vi "PeriodTuningSine.vi"(10 "cfspont":dbl, 11 "cf_right":dbl) -> (0 "Negwave":dbl, 1 "Postwave":dbl, 2 "Period":dbl, 3 "Phase reset":dbl)   [LabVIEW 2016]
uses:
  <vilib>/measure/NI_MABase.lvlib
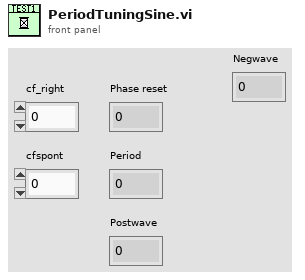
[diagram p1: front panel]
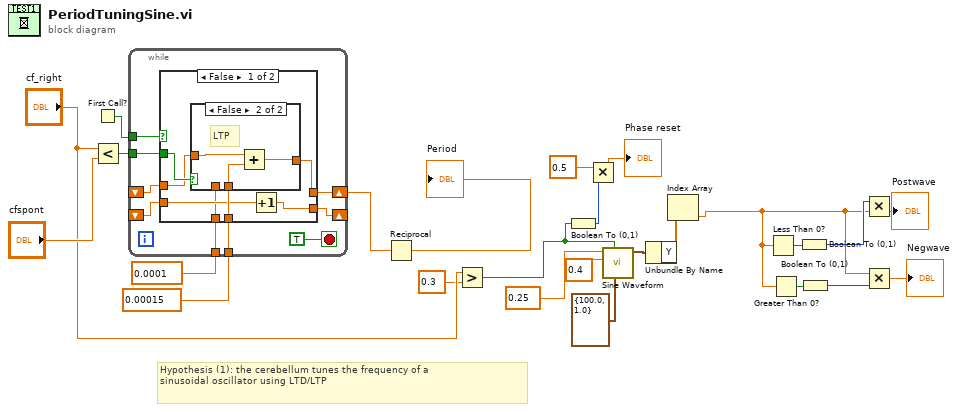
[diagram p0: block diagram]
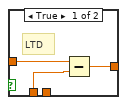
[diagram p2: hidden frame]
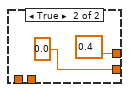
[diagram p3: hidden frame]
diagram:
  # "Hypothesis (1): the cerebellum tunes the frequency of a\nsinusoidal oscillator using LTD/LTP"
  n1 = First Call?() -> (First Call?: T/F=w11:bool)
  n2 = Less?(x="cf_right", y="cfspont") -> (x < y?=w10:bool)
  n3 = while {
    tunnel: w10 -> [w34]
    shift-right: [w31] -> w14
    shift-left: _ -> [w30]
    tunnel: w11 -> [w32]
    tunnel: 0.00015 ("y") -> [w29]
    shift-right: [w28] -> _
    shift-left: _ -> [w27]
    tunnel: 0.0001 ("y") -> [w26]
    stop <- TRUE stop-if-true
    n4 = case shown="False" w32 {
      tunnel: w34 -> [w41 _]
      tunnel: [w38 0.4] -> w31
      tunnel: w30 -> [w40 _]
      tunnel: w29 -> [w39 _]
      tunnel: [w37 0.0] -> w28
      tunnel: w27 -> [w36 _]
      tunnel: w26 -> [w35 _]
      frame False {
        n5 = case shown="False" w41 {
          tunnel: w40 -> [w44 w46]
          tunnel: w39 -> [_ w47]
          tunnel: [w43 w45] -> w38
          tunnel: w35 -> [w42 _]
          frame True {
            # "LTD"
            n6 = Subtract(x=w44, y=w42) -> (x-y=w43:dbl)
          }
          frame False {
            # "LTP"
            n7 = Add(x=w46, y=w47) -> (x+y=w45:dbl)
          }
        }
        n8 = Increment(x=w36) -> (x+1=w37:dbl)
      }
      frame True {
      }
    }
  }
  n9 = Reciprocal(x=w14) -> (1/x=→"Period":dbl)
  n10 = Greater?(x="cf_right", y=0.3) -> (0:w1:bool)
  n11 = Boolean To (0,1)(Boolean=w1) -> (0, 1=w21:i16)
  n12 = Multiply(x=0.5, y=w21) -> (x*y=→"Phase reset":dbl)
  n13 = call <vilib>:"Sine Waveform.vi"("sampling info"=cluster{"Fs":dbl, "#s":dbl} {"Fs"=100.0, "#s"=1.0}, "reset signal"=w1, "amplitude"=0.4, "frequency"=0.25) -> ("signal out"=w17:waveform(dbl))  [unwired: 6 in, 1 out]
  n14 = Unbundle By Name(w17) -> ("Y"=w18:dbl[])
  n15 = Index Array(array=w18) -> (element=w3:dbl)  [unwired: 1 in]
  n16 = Less Than 0?(x=w3) -> (x < 0?=w8:bool)
  n17 = Greater Than 0?(x=w3) -> (x > 0?=w5:bool)
  n18 = Boolean To (0,1)(Boolean=w8) -> (0, 1=w6:i16)
  n19 = Boolean To (0,1)(Boolean=w5) -> (0, 1=w4:i16)
  n20 = Multiply(x=w6, y=w3) -> (x*y=→"Postwave":dbl)
  n21 = Multiply(x=w3, y=w4) -> (x*y=→"Negwave":dbl)
